vi "WriteMultipleDataToImage.vi"(0 "DataProcessor in":refnum<class "DataProcessor.lvclass">, 5 "Image In":T1, 7 "Keys":string[](array[string]), 9 "Values":dbl[](array[numeric]), 11 "error in (no error)":errorcluster, 12 "width (-)":i16=4) -> (4 "DataProcessor out":refnum<class "DataProcessor.lvclass">, 6 "Image Out":T1, 15 "error out":errorcluster)   [LabVIEW 2020, in "DataProcessor.lvlib" / "DataProcessor.lvclass"]
uses:
  DataProcessor.lvclass
  <vilib>/vision/Image Controls.llb/IMAQ Image.ctl
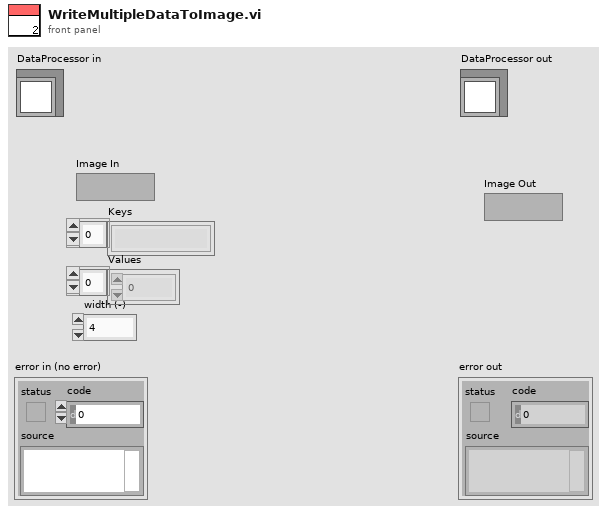
[diagram p1: front panel]
types:
  T1 = typedef "IMAQ Image.ctl" = refnum<image>
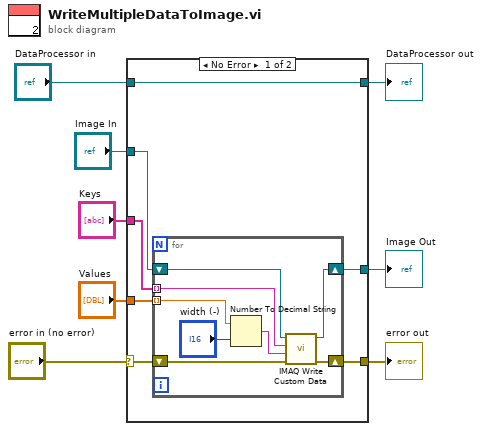
[diagram p0: block diagram]
diagram:
  n1 = case shown="No Error" "error in (no error)" {
    selector: "error in (no error)" -> [w14 w26]
    tunnel: [w13 w26] -> w3
    tunnel: [w15 w25] -> w2
    tunnel: "DataProcessor in" -> [w15 w25]
    tunnel: "Image In" -> [w12 w24]
    tunnel: "Values" -> [w9 _]
    tunnel: "Keys" -> [w10 _]
    tunnel: [w11 w24] -> w5
    frame No Error {
      n2 = for {
        tunnel: w10 -> [w18] mode=indexing
        tunnel: w9 -> [w17] mode=indexing
        shift-right: [w22] -> w13
        shift-left: w14 -> [w23]
        shift-right: [w20] -> w11
        shift-left: w12 -> [w21]
        n3 = Number To Decimal String(number=w17, width (-)="width (-)") -> (decimal integer string=w19:string)
        n4 = call "IMAQ Write Custom Data"("error in (no error)"=w23, "Custom Data In"=w19, "Key"=w18, "Image"=w21) -> ("error out"=w22:errorcluster, "Image Out"=w20:T1)  [unwired: 6 in]
      }
    }
    frame Error {
    }
  }
  "error out" <- w3
  "DataProcessor out" <- w2
  "Image Out" <- w5
